vi "Do.vi"(8 "error in (no error)":errorcluster, 10 "Actor in":refnum<class "Actor.lvclass">, 11 "Forward Direct Message Msg":refnum<class "Forward Direct Message Msg.lvclass">) -> (0 "error out":errorcluster, 2 "Actor out":refnum<class "Actor.lvclass">)   [LabVIEW 2015, in "Chat Window Model.lvlib" / "Forward Direct Message Msg.lvclass"]
doc: "This VI delivers the message to the actor by calling the appropriate method(s) on the actor."
uses:
  Forward Direct Message Msg.lvclass
  <vilib>/ActorFramework/Actor/Actor.lvclass
  Chat Window Model/Chat Window Model.lvclass
  Chat Window UI Controller/Chat Window UI Controller Messages/Direct Message Msg/Direct Message Msg.lvclass/Direct Message Msg.ctl
  Chat Window UI Controller/Chat Window UI Controller Messages/Direct Message Msg/Direct Message Msg.lvclass
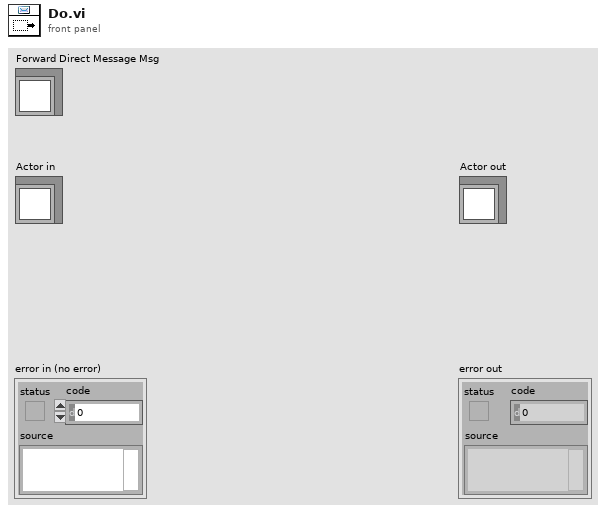
[diagram p1: front panel]
types:
  T1 = typedef "Message Control.ctl" = cluster{"From":string, "To":string, "Message":string}
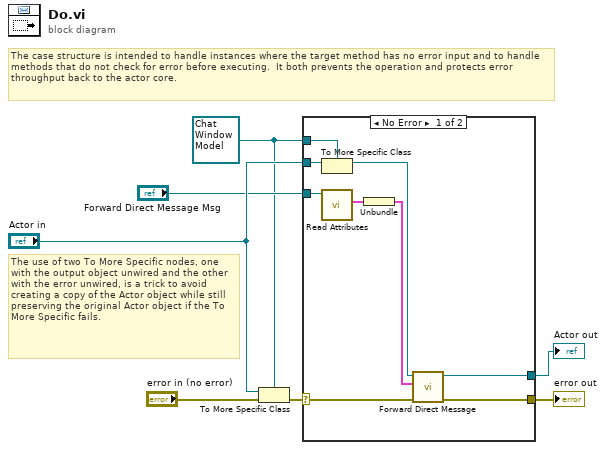
[diagram p0: block diagram]
diagram:
  w2 = refnum<class "Chat Window Model.lvclass"> refnum ("Actor in")
  # "The use of two To More Specific nodes, one with the output object unwired and the other with the error unwired, is a trick to avoid creating a copy of the Actor object while still preserving the original Actor object if the To More Specific fails."
  # "The case structure is intended to handle instances where the target method has no error input and to handle methods that do not check for error before executing.  It both prevents the operation and protects error throughput back to the actor core."
  n1 = To More Specific Class(target class=w2, reference="Actor in", error in="error in (no error)") -> (error out=w1:errorcluster)  [unwired: 1 out]
  n2 = case shown="No Error" w1 {
    selector: w1 -> [w14 w18]
    tunnel: [w16 w18] -> w7
    tunnel: [w15 w17] -> w6
    tunnel: "Actor in" -> [w13 w17]
    tunnel: w2 -> [w12 _]
    tunnel: "Forward Direct Message Msg" -> [w9 _]
    frame No Error {
      n3 = To More Specific Class(target class=w12, reference=w13) -> (specific class reference=w11:refnum<class "Chat Window Model.lvclass">)  [unwired: 1 in, 1 out]
      n4 = call "Read Attributes.vi"("Direct Message Msg"=w9) -> ("Payload"=w10:cluster{"Message":T1})  [unwired: 10 in]
      n5 = Unbundle(w10) -> ("Message"=w8:T1)
      n6 = call "Forward Direct Message.vi"("error in (no error)"=w14, "Message"=w8, "Chat Window Model in"=w11) -> ("error out"=w16:errorcluster, "Chat Window Model out"=w15:refnum<class "Chat Window Model.lvclass">)  [unwired: 7 in]
    }
    frame Error {
      # "If type check fails, pass the original object out again."
    }
  }
  "error out" <- w7
  "Actor out" <- w6
